vi "RF_Sig_Gen.vi"(0 "Signal Generator Control":T2={"Frequency (GHz)"=2.809, "RF Power (dBm)"=-120.0, "RF ON/OFF"=FALSE} {"RF Power (dBm)" min=-120.0 max=20.0 step=0.02 format="%.2g"; "Frequency (GHz)" min=0.6 max=3.0 step=0.001 format="%#_9g"}, 9 "Timeout mS":i32=100, 11 "error in":errorcluster) -> (4 "Signal Generator Status":T1={"Frequency (GHz)"=2809000000.0, "RF Power (dBm)"=-120.0, "RF Power"=FALSE} {"RF Power (dBm)" format="%.2g"}, 15 "Sig Gen Errors":errorcluster)   [LabVIEW 2012]
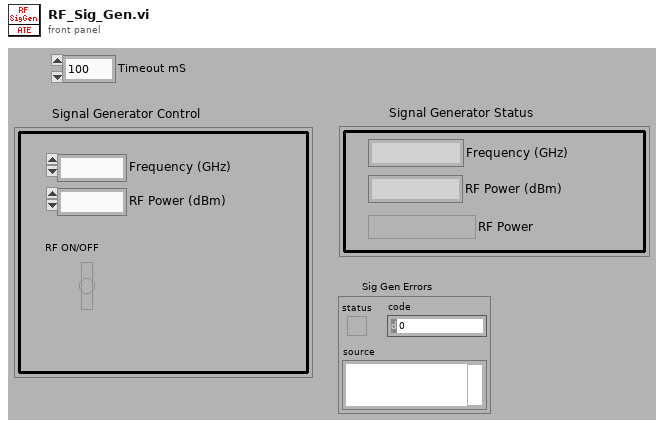
[diagram p1: front panel]
types:
  T1 = cluster{"Frequency (GHz)":dbl, "RF Power (dBm)":dbl, "RF Power":bool}
  T2 = cluster{"Frequency (GHz)":dbl, "RF Power (dBm)":dbl, "RF ON/OFF":bool}
  T3 = enum16{"N1911A", "Siggen", "34980a", "E4418B", "Rvp8"}
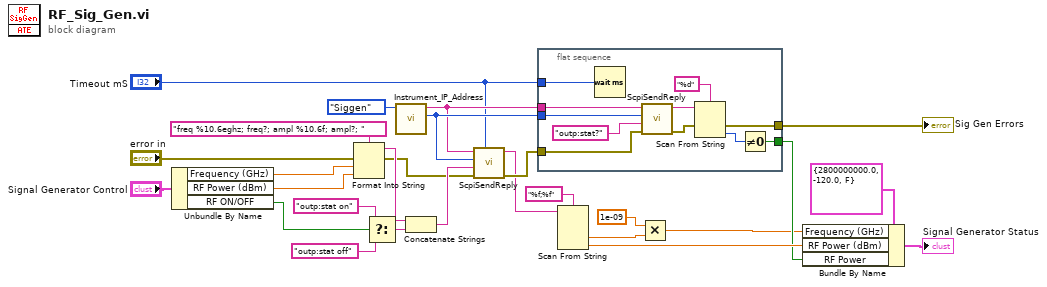
[diagram p0: block diagram]
diagram:
  n1 = Unbundle By Name("Signal Generator Control") -> ("Frequency (GHz)"=w13:dbl, "RF Power (dBm)"=w11:dbl, "RF ON/OFF"=w12:bool)
  n2 = Format Into String(format string="freq %10.6eghz; freq?; ampl %10.6f; ampl?; ", error in="error in", w13, w11) -> (resulting string=w23:string, error out=w15:errorcluster)  [unwired: 1 in]
  n3 = Select(t="outp:stat on" ("format string"), s=w12, f="outp:stat off" ("format string")) -> (s? t:f=w24:string)
  n4 = call "Instrument_IP_Address.vi"("Instrument"=T3."Siggen") -> ("Port"=w20:u16, "IP Address"=w18:string)  [unwired: 9 in]
  n5 = Concatenate Strings(w23, w24) -> (w22:string)
  n6 = call "ScpiSendReply.vi"("TCP Timeout mS"="Timeout mS", "error in (no error)"=w15, "Command"=w22, "TCP port"=w20, "IP Address"=w18) -> ("Error out"=w19:errorcluster, "Reply"=w17:string)  [unwired: 4 in]
  n7 = flat-sequence {
    tunnel: w19 -> [w32]
    tunnel: w18 -> [w37]
    tunnel: w20 -> [w36]
    tunnel: [w30] -> w8
    tunnel: [w29] -> w10
    tunnel: "Timeout mS" -> [w28]
    frame #0 {
      n8 = Wait (ms)(milliseconds to wait=w28) -> ()  [unwired: 1 out]
      n9 = call "ScpiSendReply.vi"("error in (no error)"=w32, "Command"="outp:stat?", "TCP port"=w36, "IP Address"=w37) -> ("Error out"=w31:errorcluster, "Reply"=w33:string)  [unwired: 5 in]
      n10 = Scan From String(format string="%d", input string=w33, error in=w31) -> (error out=w29:errorcluster, output 1=w34:i32)  [unwired: 2 in, 2 out]
      n11 = Not Equal To 0?(x=w34) -> (x != 0?=w30:bool)
    }
  }
  n12 = Scan From String(format string="%f;%f", input string=w17) -> (output 1=w2:dbl, output 2=w9:dbl)  [unwired: 4 in, 3 out]
  n13 = Multiply(x=1e-09, y=w2) -> (x*y=w1:dbl)
  n14 = Bundle By Name(cluster=T1 {"Frequency (GHz)"=2800000000.0, "RF Power (dBm)"=-120.0, "RF Power"=FALSE} ("Signal Generator Status"), "Frequency (GHz)"=w1, "RF Power (dBm)"=w9, "RF Power"=w8) -> (→"Signal Generator Status":T1)
  "Sig Gen Errors" <- w10
